vi "3. ControlRealTimeACCESS.vi"() -> ()   [LabVIEW 2011]
panel:
  out "Iteration #":i32
  out "mote111":cluster{dbl, dbl}
  out "mote110":cluster{dbl, dbl}
  out "mote109":cluster{dbl, dbl}
  out "mote12":cluster{dbl, dbl}
  out "mote11":cluster{dbl, dbl}
  out "mote8":cluster{dbl, dbl}
  out "mote7":cluster{dbl, dbl}
  out "mote6":cluster{dbl, dbl}
  out "mote5":cluster{dbl, dbl}
  out "mote3":cluster{dbl, dbl}
  out "mote2":cluster{dbl, dbl}
  out "mote4":cluster{dbl, dbl, dbl, dbl}
  out "mote1":cluster{dbl, dbl, dbl, dbl}
  in  "HVAC Testbed":T1(tab)
  out "Motion":bool
  out "CO2":string
  out "Temp":string
  out "Temp":string
  out "CO2":string
  out "Motion":bool
  out "Temp":string
  out "CO2":string
  out "Motion":bool
  out "CO2":string
  out "Temp":string
  out "Motion":bool
  out "Outside temp":dbl(slide) scale=-20.0..40.0
  in  "Heating Valve":u64(slide) scale=0.0..100.0
  in  "Cooling Valve":u64(slide) scale=0.0..100.0
  in  "Fresh Air Valve":u64(slide) scale=0.0..100.0
  out "Temp":string
  out "CO2":string
  out "Motion":bool
  out "CO2":dbl(graph)
  out "Temperature":dbl(graph)
  out "CO2":dbl(graph)
  out "Temperature":dbl(graph)
  in  "Heating Valve":u64(slide) scale=0.0..100.0
  in  "Cooling Valve":u64(slide) scale=0.0..100.0
  in  "Fresh Air Valve":u64(slide) scale=0.0..100.0
  out "Occupancy":dbl
  out "Temp":string
  out "CO2":string
  out "Motion":bool
  out "Light":dbl(slide) scale=0.0..100.0
  in  "12":bool
  in  "11":bool
  in  "4":bool
  in  "111":bool
  in  "110":bool
  in  "109":bool
  in  "8":bool
  in  "7":bool
  in  "5":bool
  in  "4":bool
  in  "3":bool
  in  "1":bool
  in  "6":bool
  in  "2":bool
  out "Humidity":dbl(slide) scale=0.0..100.0
  out "Temperature":dbl(slide) scale=0.0..100.0
  out "CO2 Meter":dbl(knob) scale=0.0..800.0
  out "Selected Mote":string
  out "CO2":dbl(graph)
  out "Temperature":dbl(graph)
  in  "Heating Valve":u64(slide) scale=0.0..100.0
  in  "Cooling Valve":u64(slide) scale=0.0..100.0
  in  "Fresh Air Valve":u64(slide) scale=0.0..100.0
  out "Temp":string
  out "CO2":string
  out "Motion":bool
  in  "HVAC System IP Address":string(combo)="130.237.50.30"
  in  "Password":string
  in  "Username":string
  out "Access to HVAC Msg":errorcluster={"status"=FALSE, "code"=0, "source"="Please Wait ..."}
  # "Actuation"
  # "PLC Data"
  # "Selected Mote Data"
  # "PLC Data"
  # "Actuation"
  # "Actuation"
  # "PLC Data"
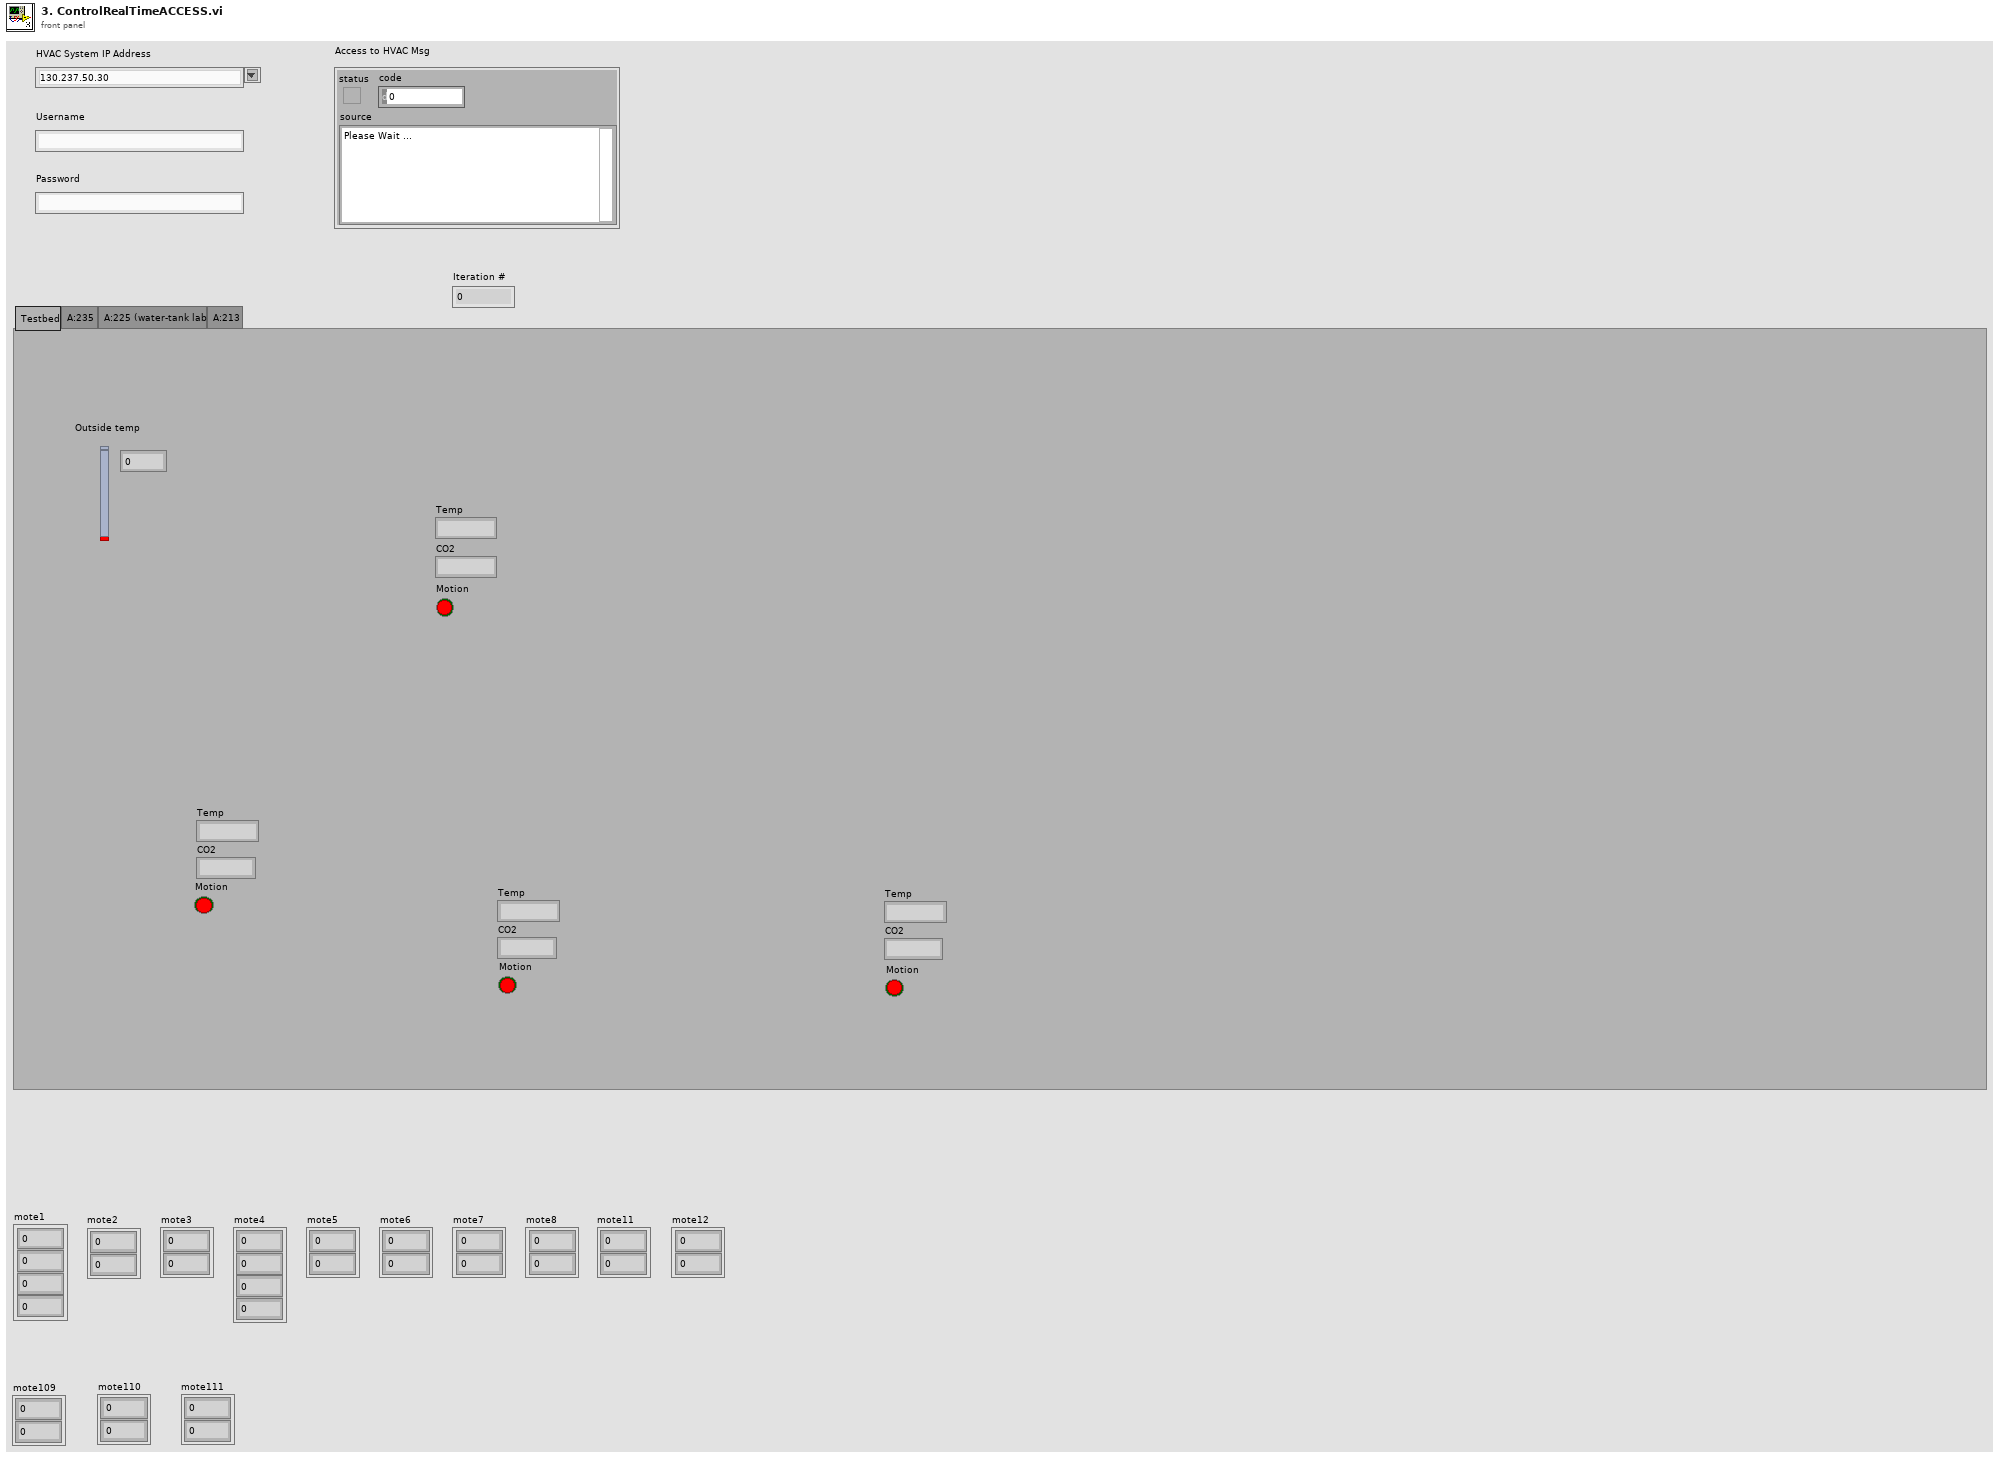
[diagram p1: front panel]
types:
  T1 = enum32{"Testbed", "A:235", "A:225 (water-tank lab)", "A:213"}
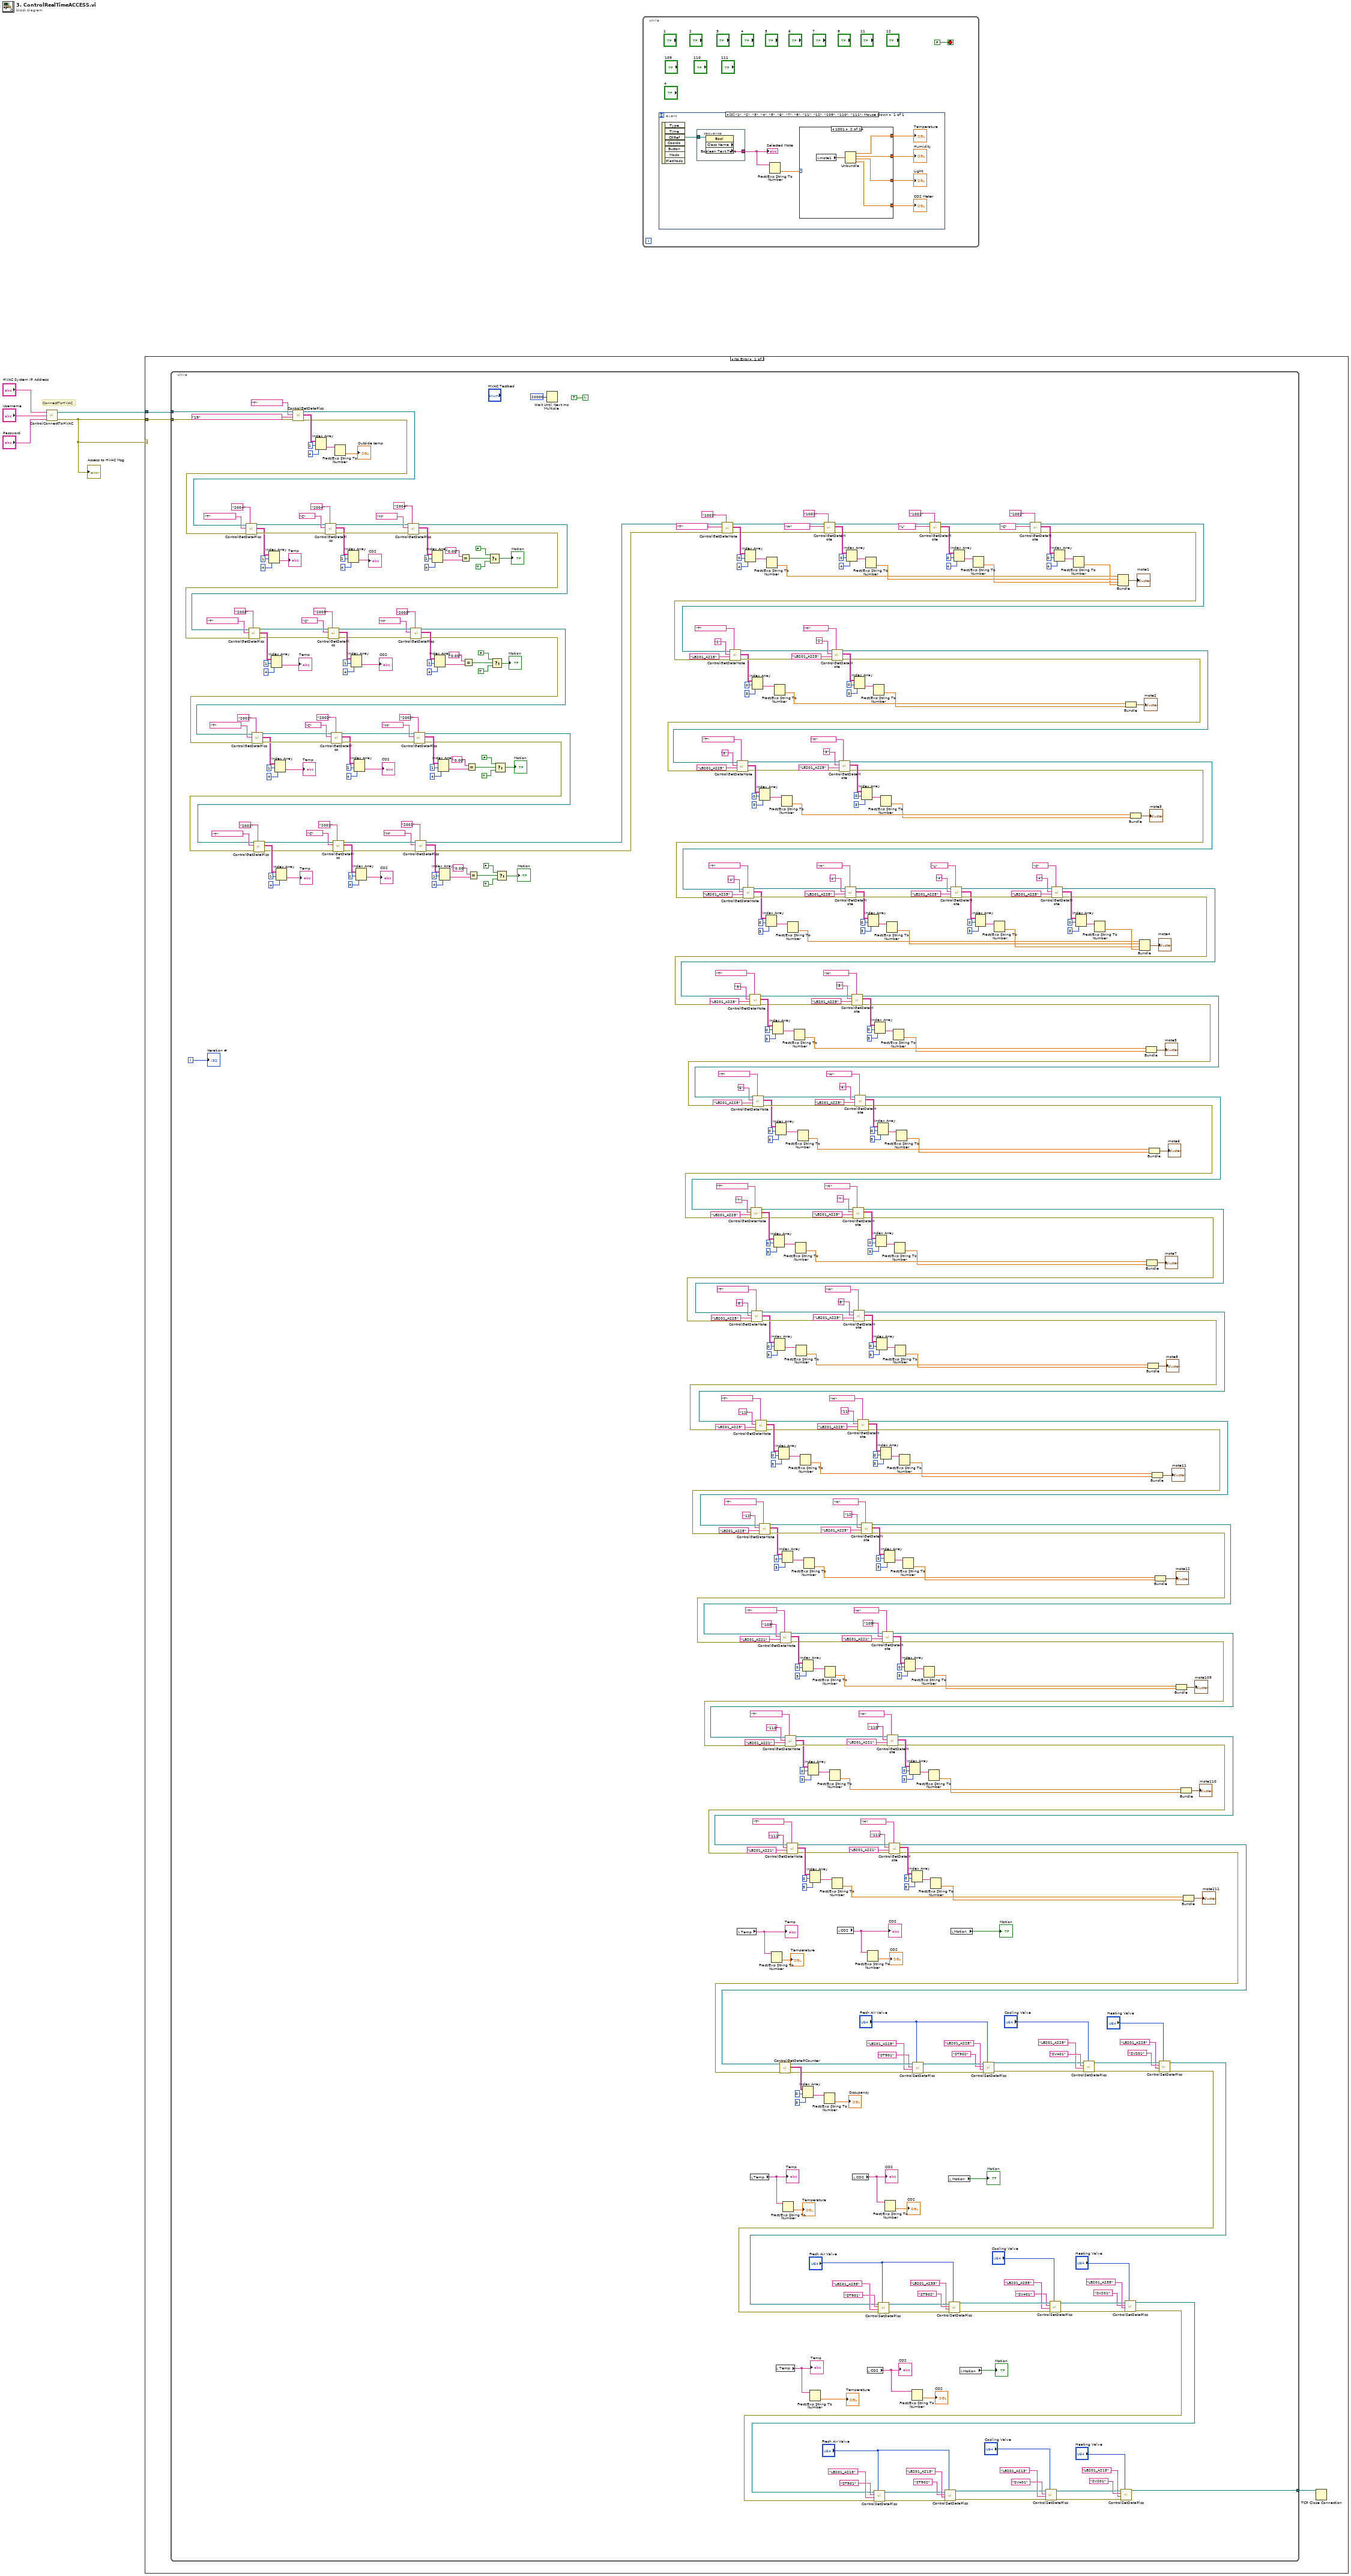
[diagram p0: block diagram]
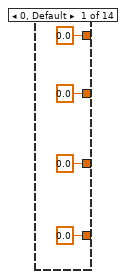
[diagram p2: hidden frame]
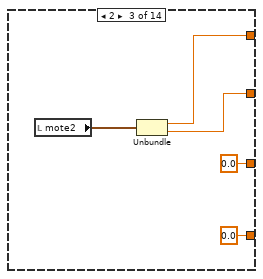
[diagram p3: hidden frame]
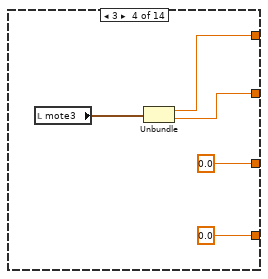
[diagram p4: hidden frame]
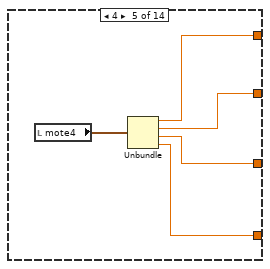
[diagram p5: hidden frame]
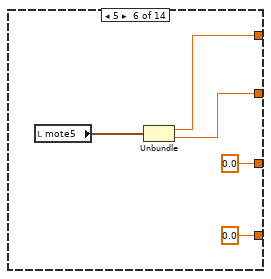
[diagram p6: hidden frame]
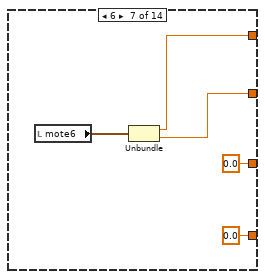
[diagram p7: hidden frame]
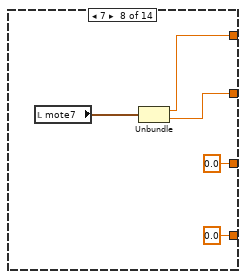
[diagram p8: hidden frame]
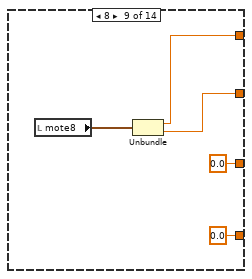
[diagram p9: hidden frame]
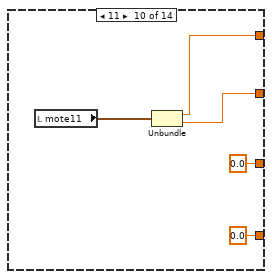
[diagram p10: hidden frame]
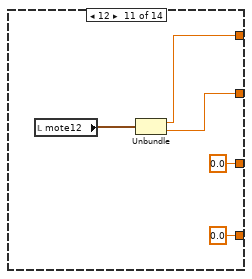
[diagram p11: hidden frame]
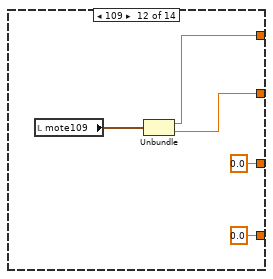
[diagram p12: hidden frame]
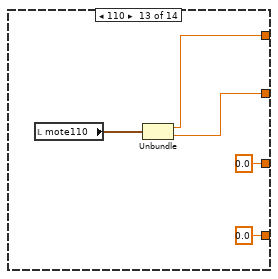
[diagram p13: hidden frame]
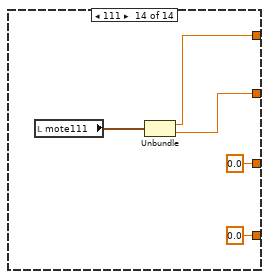
[diagram p14: hidden frame]
diagram:
  # "ConnectToHVAC"
  n1 = call "ControlConnectToHVAC.vi"("Password"="Password", "Username"="Username", "IP Address"="HVAC System IP Address") -> ("error out"=w4:errorcluster, "connection ID out"=w5:refnum<k5>)  [unwired: 1 in]
  "Access to HVAC Msg" <- w4
  n2 = case shown="No Error" w4 {
    tunnel: w5 -> [w7 _]
    tunnel: w4 -> [w8 _]
    frame No Error {
      n3 = while {
        tunnel: w7 -> [w501]
        tunnel: w8 -> [w502]
        tunnel: [w41] -> w6
        i -> [w396]
        stop <- TRUE continue-if-true
        n4 = call "ControlGetDataPlcs.vi"("error in"=w502, "signalID"="19", "dataType"="T" ("Data Type"), "connection ID in"=w501) -> ("error out"=w499:errorcluster, "output array"=w507:string[][], "connection ID out"=w500:refnum<k5>)  [unwired: 4 in]
        n5 = call "ControlGetDataPlcs.vi"("deviceID"="2004", "error in"=w499, "dataType"="T" ("Data Type"), "connection ID in"=w500) -> ("error out"=w519:errorcluster, "output array"=w514:string[][], "connection ID out"=w520:refnum<k5>)  [unwired: 4 in]
        n6 = Index Array(array=w514, index (row)=1, index (col)=4 ("disabled index (col)")) -> (element=→"Temp":string)
        n7 = Index Array(array=w507, index (row)=1, index (col)=4 ("disabled index (col)")) -> (element=w506:string)
        n8 = call "ControlGetDataPlcs.vi"("deviceID"="2004", "error in"=w519, "dataType"="C" ("Data Type"), "connection ID in"=w520) -> ("error out"=w518:errorcluster, "output array"=w509:string[][], "connection ID out"=w517:refnum<k5>)  [unwired: 4 in]
        n9 = Fract/Exp String To Number(string=w506) -> (number=→"Outside temp":dbl)  [unwired: 3 in, 1 out]
        n10 = Index Array(array=w509, index (row)=1, index (col)=4 ("disabled index (col)")) -> (element=→"CO2":string)
        n11 = call "ControlGetDataPlcs.vi"("deviceID"="2004", "error in"=w518, "dataType"="M" ("Data Type"), "connection ID in"=w517) -> ("error out"=w471:errorcluster, "output array"=w508:string[][], "connection ID out"=w472:refnum<k5>)  [unwired: 4 in]
        n12 = call "ControlGetDataPlcs.vi"("deviceID"="2003", "error in"=w471, "dataType"="T" ("Data Type"), "connection ID in"=w472) -> ("error out"=w477:errorcluster, "output array"=w482:string[][], "connection ID out"=w476:refnum<k5>)  [unwired: 4 in]
        n13 = Index Array(array=w482, index (row)=1, index (col)=4 ("disabled index (col)")) -> (element=→"Temp":string)
        n14 = call "ControlGetDataPlcs.vi"("deviceID"="2003", "error in"=w477, "dataType"="C" ("Data Type"), "connection ID in"=w476) -> ("error out"=w478:errorcluster, "output array"=w487:string[][], "connection ID out"=w479:refnum<k5>)  [unwired: 4 in]
        n15 = Index Array(array=w487, index (row)=1, index (col)=4 ("disabled index (col)")) -> (element=→"CO2":string)
        n16 = call "ControlGetDataPlcs.vi"("deviceID"="2003", "error in"=w478, "dataType"="M" ("Data Type"), "connection ID in"=w479) -> ("error out"=w448:errorcluster, "output array"=w488:string[][], "connection ID out"=w449:refnum<k5>)  [unwired: 4 in]
        n17 = call "ControlGetDataPlcs.vi"("deviceID"="2002", "error in"=w448, "dataType"="T" ("Data Type"), "connection ID in"=w449) -> ("error out"=w466:errorcluster, "output array"=w461:string[][], "connection ID out"=w467:refnum<k5>)  [unwired: 4 in]
        n18 = Index Array(array=w461, index (row)=1, index (col)=4 ("disabled index (col)")) -> (element=→"Temp":string)
        n19 = call "ControlGetDataPlcs.vi"("deviceID"="2002", "error in"=w466, "dataType"="C" ("Data Type"), "connection ID in"=w467) -> ("error out"=w465:errorcluster, "output array"=w456:string[][], "connection ID out"=w464:refnum<k5>)  [unwired: 4 in]
        n20 = Index Array(array=w456, index (row)=1, index (col)=4 ("disabled index (col)")) -> (element=→"CO2":string)
        n21 = call "ControlGetDataPlcs.vi"("deviceID"="2002", "error in"=w465, "dataType"="M" ("Data Type"), "connection ID in"=w464) -> ("error out"=w425:errorcluster, "output array"=w455:string[][], "connection ID out"=w426:refnum<k5>)  [unwired: 4 in]
        n22 = call "ControlGetDataPlcs.vi"("deviceID"="2001", "error in"=w425, "dataType"="T" ("Data Type"), "connection ID in"=w426) -> ("error out"=w431:errorcluster, "output array"=w436:string[][], "connection ID out"=w430:refnum<k5>)  [unwired: 4 in]
        n23 = Index Array(array=w436, index (row)=1, index (col)=4 ("disabled index (col)")) -> (element=→"Temp":string)
        n24 = call "ControlGetDataPlcs.vi"("deviceID"="2001", "error in"=w431, "dataType"="C" ("Data Type"), "connection ID in"=w430) -> ("error out"=w432:errorcluster, "output array"=w441:string[][], "connection ID out"=w433:refnum<k5>)  [unwired: 4 in]
        n25 = Index Array(array=w441, index (row)=1, index (col)=4 ("disabled index (col)")) -> (element=→"CO2":string)
        n26 = call "ControlGetDataPlcs.vi"("deviceID"="2001", "error in"=w432, "dataType"="M" ("Data Type"), "connection ID in"=w433) -> ("error out"=w397:errorcluster, "output array"=w442:string[][], "connection ID out"=w398:refnum<k5>)  [unwired: 4 in]
        n27 = Index Array(array=w508, index (row)=1, index (col)=4 ("disabled index (col)")) -> (element=w497:string)
        n28 = Index Array(array=w488, index (row)=1, index (col)=4 ("disabled index (col)")) -> (element=w490:string)
        n29 = Index Array(array=w455, index (row)=1, index (col)=4 ("disabled index (col)")) -> (element=w453:string)
        n30 = Index Array(array=w442, index (row)=1, index (col)=4 ("disabled index (col)")) -> (element=w444:string)
        n31 = Equal?(x="0.00", y=w497) -> (x = y?=w496:bool)
        n32 = Equal?(x="0.00", y=w490) -> (x = y?=w491:bool)
        n33 = Equal?(x="0.00", y=w453) -> (x = y?=w452:bool)
        n34 = Equal?(x="0.00", y=w444) -> (x = y?=w445:bool)
        n35 = Select(t=FALSE, s=w496, f=TRUE) -> (s? t:f=→"Motion":bool)
        n36 = Select(t=FALSE, s=w491, f=TRUE) -> (s? t:f=→"Motion":bool)
        n37 = Select(t=FALSE, s=w452, f=TRUE) -> (s? t:f=→"Motion":bool)
        n38 = Select(t=FALSE, s=w445, f=TRUE) -> (s? t:f=→"Motion":bool)
        n39 = Wait Until Next ms Multiple(millisecond multiple=u32 20000) -> ()  [unwired: 1 out]
        n40 = call "ControlGetDataMote.vi"("deviceID"="1001" ("Node ID"), "error in"=w397, "dataType"="T" ("Data Type"), "connection ID in"=w398) -> ("error out"=w400:errorcluster, "output array"=w405:string[][], "connection ID out"=w399:refnum<k5>)  [unwired: 5 in]
        n41 = local read "Temp"() -> (w83:string)
        "Temp" <- w83
        n42 = Index Array(array=w405, index (row)=0, index (col)=4 ("disabled index (col)")) -> (element=w395:string)
        n43 = local read "Temp"() -> (w78:string)
        "Temp" <- w78
        n44 = Fract/Exp String To Number(string=w395) -> (number=w392:dbl)  [unwired: 3 in, 1 out]
        n45 = Fract/Exp String To Number(string=w83) -> (number=→"Temperature":dbl)  [unwired: 3 in, 1 out]
        n46 = local read "Temp"() -> (w59:string)
        "Temp" <- w59
        n47 = Fract/Exp String To Number(string=w78) -> (number=→"Temperature":dbl)  [unwired: 3 in, 1 out]
        n48 = Fract/Exp String To Number(string=w59) -> (number=→"Temperature":dbl)  [unwired: 3 in, 1 out]
        n49 = call "ControlGetDataMote.vi"("deviceID"="1001" ("Node ID"), "error in"=w400, "dataType"="H" ("Data Type"), "connection ID in"=w399) -> ("error out"=w401:errorcluster, "output array"=w410:string[][], "connection ID out"=w402:refnum<k5>)  [unwired: 5 in]
        n50 = local read "CO2"() -> (w82:string)
        "CO2" <- w82
        n51 = Index Array(array=w410, index (row)=0, index (col)=4 ("disabled index (col)")) -> (element=w394:string)
        n52 = local read "CO2"() -> (w77:string)
        "CO2" <- w77
        n53 = Fract/Exp String To Number(string=w394) -> (number=w391:dbl)  [unwired: 3 in, 1 out]
        n54 = Fract/Exp String To Number(string=w82) -> (number=→"CO2":dbl)  [unwired: 3 in, 1 out]
        n55 = local read "CO2"() -> (w58:string)
        "CO2" <- w58
        n56 = Fract/Exp String To Number(string=w77) -> (number=→"CO2":dbl)  [unwired: 3 in, 1 out]
        n57 = Fract/Exp String To Number(string=w58) -> (number=→"CO2":dbl)  [unwired: 3 in, 1 out]
        n58 = call "ControlGetDataMote.vi"("deviceID"="1001" ("Node ID"), "error in"=w401, "dataType"="L" ("Data Type"), "connection ID in"=w402) -> ("error out"=w382:errorcluster, "output array"=w411:string[][], "connection ID out"=w385:refnum<k5>)  [unwired: 5 in]
        n59 = local read "Motion"() -> (→"Motion":bool)
        n60 = local read "Motion"() -> (→"Motion":bool)
        n61 = Index Array(array=w411, index (row)=0, index (col)=4 ("disabled index (col)")) -> (element=w393:string)
        n62 = local read "Motion"() -> (→"Motion":bool)
        n63 = Fract/Exp String To Number(string=w393) -> (number=w390:dbl)  [unwired: 3 in, 1 out]
        n64 = call "ControlGetDataMote.vi"("deviceID"="1001" ("Node ID"), "error in"=w382, "dataType"="C" ("Data Type"), "connection ID in"=w385) -> ("error out"=w305:errorcluster, "output array"=w386:string[][], "connection ID out"=w306:refnum<k5>)  [unwired: 5 in]
        n65 = call "ControlGetDataMote.vi"("deviceID"="T" ("Data Type"), "error in"=w305, "signalID"="LB201_A225" ("Location"), "dataType"="2" ("Node ID"), "connection ID in"=w306) -> ("error out"=w370:errorcluster, "output array"=w367:string[][], "connection ID out"=w371:refnum<k5>)  [unwired: 4 in]
        n66 = Index Array(array=w367, index (row)=0, index (col)=3 ("disabled index (col)")) -> (element=w378:string)
        n67 = Fract/Exp String To Number(string=w378) -> (number=w380:dbl)  [unwired: 3 in, 1 out]
        n68 = call "ControlGetDataMote.vi"("deviceID"="H" ("Data Type"), "error in"=w370, "signalID"="LB201_A225" ("Location"), "dataType"="2" ("Node ID"), "connection ID in"=w371) -> ("error out"=w301:errorcluster, "output array"=w364:string[][], "connection ID out"=w302:refnum<k5>)  [unwired: 4 in]
        n69 = call "ControlGetDataMote.vi"("deviceID"="T" ("Data Type"), "error in"=w301, "signalID"="LB201_A225" ("Location"), "dataType"="3" ("Node ID"), "connection ID in"=w302) -> ("error out"=w357:errorcluster, "output array"=w360:string[][], "connection ID out"=w356:refnum<k5>)  [unwired: 4 in]
        n70 = Index Array(array=w360, index (row)=0, index (col)=3 ("disabled index (col)")) -> (element=w349:string)
        n71 = Fract/Exp String To Number(string=w349) -> (number=w347:dbl)  [unwired: 3 in, 1 out]
        n72 = call "ControlGetDataMote.vi"("deviceID"="H" ("Data Type"), "error in"=w357, "signalID"="LB201_A225" ("Location"), "dataType"="3" ("Node ID"), "connection ID in"=w356) -> ("error out"=w303:errorcluster, "output array"=w363:string[][], "connection ID out"=w304:refnum<k5>)  [unwired: 4 in]
        n73 = call "ControlGetDataMote.vi"("deviceID"="T" ("Data Type"), "error in"=w303, "signalID"="LB201_A225" ("Location"), "dataType"="4" ("Node ID"), "connection ID in"=w304) -> ("error out"=w318:errorcluster, "output array"=w313:string[][], "connection ID out"=w319:refnum<k5>)  [unwired: 4 in]
        n74 = Index Array(array=w313, index (row)=0, index (col)=3 ("disabled index (col)")) -> (element=w329:string)
        n75 = Fract/Exp String To Number(string=w329) -> (number=w332:dbl)  [unwired: 3 in, 1 out]
        n76 = call "ControlGetDataMote.vi"("deviceID"="H" ("Data Type"), "error in"=w318, "signalID"="LB201_A225" ("Location"), "dataType"="4" ("Node ID"), "connection ID in"=w319) -> ("error out"=w317:errorcluster, "output array"=w308:string[][], "connection ID out"=w316:refnum<k5>)  [unwired: 4 in]
        n77 = Index Array(array=w364, index (row)=0, index (col)=3 ("disabled index (col)")) -> (element=w379:string)
        n78 = Index Array(array=w363, index (row)=0, index (col)=3 ("disabled index (col)")) -> (element=w348:string)
        n79 = Index Array(array=w308, index (row)=0, index (col)=3 ("disabled index (col)")) -> (element=w330:string)
        n80 = Fract/Exp String To Number(string=w379) -> (number=w381:dbl)  [unwired: 3 in, 1 out]
        n81 = Fract/Exp String To Number(string=w348) -> (number=w346:dbl)  [unwired: 3 in, 1 out]
        n82 = Fract/Exp String To Number(string=w330) -> (number=w333:dbl)  [unwired: 3 in, 1 out]
        n83 = call "ControlGetDataMote.vi"("deviceID"="L" ("Data Type"), "error in"=w317, "signalID"="LB201_A225" ("Location"), "dataType"="4" ("Node ID"), "connection ID in"=w316) -> ("error out"=w345:errorcluster, "output array"=w307:string[][], "connection ID out"=w342:refnum<k5>)  [unwired: 4 in]
        n84 = Index Array(array=w307, index (row)=0, index (col)=3 ("disabled index (col)")) -> (element=w331:string)
        n85 = Fract/Exp String To Number(string=w331) -> (number=w334:dbl)  [unwired: 3 in, 1 out]
        n86 = call "ControlGetDataMote.vi"("deviceID"="C" ("Data Type"), "error in"=w345, "signalID"="LB201_A225" ("Location"), "dataType"="4" ("Node ID"), "connection ID in"=w342) -> ("error out"=w189:errorcluster, "output array"=w341:string[][], "connection ID out"=w190:refnum<k5>)  [unwired: 4 in]
        n87 = call "ControlGetDataMote.vi"("deviceID"="T" ("Data Type"), "error in"=w189, "signalID"="LB201_A225" ("Location"), "dataType"="5" ("Node ID"), "connection ID in"=w190) -> ("error out"=w292:errorcluster, "output array"=w295:string[][], "connection ID out"=w291:refnum<k5>)  [unwired: 4 in]
        n88 = Index Array(array=w295, index (row)=0, index (col)=3 ("disabled index (col)")) -> (element=w284:string)
        n89 = Fract/Exp String To Number(string=w284) -> (number=w282:dbl)  [unwired: 3 in, 1 out]
        n90 = call "ControlGetDataMote.vi"("deviceID"="H" ("Data Type"), "error in"=w292, "signalID"="LB201_A225" ("Location"), "dataType"="5" ("Node ID"), "connection ID in"=w291) -> ("error out"=w185:errorcluster, "output array"=w298:string[][], "connection ID out"=w186:refnum<k5>)  [unwired: 4 in]
        n91 = call "ControlGetDataMote.vi"("deviceID"="T" ("Data Type"), "error in"=w185, "signalID"="LB201_A225" ("Location"), "dataType"="6" ("Node ID"), "connection ID in"=w186) -> ("error out"=w269:errorcluster, "output array"=w266:string[][], "connection ID out"=w270:refnum<k5>)  [unwired: 4 in]
        n92 = Index Array(array=w266, index (row)=0, index (col)=3 ("disabled index (col)")) -> (element=w277:string)
        n93 = Fract/Exp String To Number(string=w277) -> (number=w279:dbl)  [unwired: 3 in, 1 out]
        n94 = call "ControlGetDataMote.vi"("deviceID"="H" ("Data Type"), "error in"=w269, "signalID"="LB201_A225" ("Location"), "dataType"="6" ("Node ID"), "connection ID in"=w270) -> ("error out"=w182:errorcluster, "output array"=w263:string[][], "connection ID out"=w183:refnum<k5>)  [unwired: 4 in]
        n95 = call "ControlGetDataMote.vi"("deviceID"="T" ("Data Type"), "error in"=w182, "signalID"="LB201_A225" ("Location"), "dataType"="7" ("Node ID"), "connection ID in"=w183) -> ("error out"=w256:errorcluster, "output array"=w259:string[][], "connection ID out"=w255:refnum<k5>)  [unwired: 4 in]
        n96 = Index Array(array=w259, index (row)=0, index (col)=3 ("disabled index (col)")) -> (element=w248:string)
        n97 = Fract/Exp String To Number(string=w248) -> (number=w246:dbl)  [unwired: 3 in, 1 out]
        n98 = call "ControlGetDataMote.vi"("deviceID"="H" ("Data Type"), "error in"=w256, "signalID"="LB201_A225" ("Location"), "dataType"="7" ("Node ID"), "connection ID in"=w255) -> ("error out"=w179:errorcluster, "output array"=w262:string[][], "connection ID out"=w180:refnum<k5>)  [unwired: 4 in]
        n99 = call "ControlGetDataMote.vi"("deviceID"="T" ("Data Type"), "error in"=w179, "signalID"="LB201_A225" ("Location"), "dataType"="8" ("Node ID"), "connection ID in"=w180) -> ("error out"=w233:errorcluster, "output array"=w230:string[][], "connection ID out"=w234:refnum<k5>)  [unwired: 4 in]
        n100 = Index Array(array=w230, index (row)=0, index (col)=3 ("disabled index (col)")) -> (element=w241:string)
        n101 = Fract/Exp String To Number(string=w241) -> (number=w243:dbl)  [unwired: 3 in, 1 out]
        n102 = call "ControlGetDataMote.vi"("deviceID"="H" ("Data Type"), "error in"=w233, "signalID"="LB201_A225" ("Location"), "dataType"="8" ("Node ID"), "connection ID in"=w234) -> ("error out"=w139:errorcluster, "output array"=w227:string[][], "connection ID out"=w140:refnum<k5>)  [unwired: 4 in]
        n103 = call "ControlGetDataMote.vi"("deviceID"="T" ("Data Type"), "error in"=w139, "signalID"="LB201_A225" ("Location"), "dataType"="11" ("Node ID"), "connection ID in"=w140) -> ("error out"=w220:errorcluster, "output array"=w223:string[][], "connection ID out"=w219:refnum<k5>)  [unwired: 4 in]
        n104 = Index Array(array=w223, index (row)=0, index (col)=3 ("disabled index (col)")) -> (element=w212:string)
        n105 = Fract/Exp String To Number(string=w212) -> (number=w210:dbl)  [unwired: 3 in, 1 out]
        n106 = call "ControlGetDataMote.vi"("deviceID"="H" ("Data Type"), "error in"=w220, "signalID"="LB201_A225" ("Location"), "dataType"="11" ("Node ID"), "connection ID in"=w219) -> ("error out"=w137:errorcluster, "output array"=w226:string[][], "connection ID out"=w138:refnum<k5>)  [unwired: 4 in]
        n107 = call "ControlGetDataMote.vi"("deviceID"="T" ("Data Type"), "error in"=w137, "signalID"="LB201_A225" ("Location"), "dataType"="12" ("Node ID"), "connection ID in"=w138) -> ("error out"=w197:errorcluster, "output array"=w194:string[][], "connection ID out"=w198:refnum<k5>)  [unwired: 4 in]
        n108 = Index Array(array=w194, index (row)=0, index (col)=3 ("disabled index (col)")) -> (element=w205:string)
        n109 = Fract/Exp String To Number(string=w205) -> (number=w207:dbl)  [unwired: 3 in, 1 out]
        n110 = call "ControlGetDataMote.vi"("deviceID"="H" ("Data Type"), "error in"=w197, "signalID"="LB201_A225" ("Location"), "dataType"="12" ("Node ID"), "connection ID in"=w198) -> ("error out"=w114:errorcluster, "output array"=w191:string[][], "connection ID out"=w115:refnum<k5>)  [unwired: 4 in]
        n111 = call "ControlGetDataMote.vi"("deviceID"="T" ("Data Type"), "error in"=w114, "signalID"="LB201_A221" ("Location"), "dataType"="109" ("Node ID"), "connection ID in"=w115) -> ("error out"=w172:errorcluster, "output array"=w175:string[][], "connection ID out"=w171:refnum<k5>)  [unwired: 4 in]
        n112 = Index Array(array=w175, index (row)=0, index (col)=3 ("disabled index (col)")) -> (element=w164:string)
        n113 = Fract/Exp String To Number(string=w164) -> (number=w162:dbl)  [unwired: 3 in, 1 out]
        n114 = Index Array(array=w298, index (row)=0, index (col)=3 ("disabled index (col)")) -> (element=w283:string)
        n115 = Index Array(array=w262, index (row)=0, index (col)=3 ("disabled index (col)")) -> (element=w247:string)
        n116 = Index Array(array=w227, index (row)=0, index (col)=3 ("disabled index (col)")) -> (element=w242:string)
        n117 = Index Array(array=w263, index (row)=0, index (col)=3 ("disabled index (col)")) -> (element=w278:string)
        n118 = Index Array(array=w226, index (row)=0, index (col)=3 ("disabled index (col)")) -> (element=w211:string)
        n119 = call "ControlGetDataMote.vi"("deviceID"="H" ("Data Type"), "error in"=w172, "signalID"="LB201_A221" ("Location"), "dataType"="109" ("Node ID"), "connection ID in"=w171) -> ("error out"=w112:errorcluster, "output array"=w178:string[][], "connection ID out"=w113:refnum<k5>)  [unwired: 4 in]
        n120 = call "ControlGetDataMote.vi"("deviceID"="T" ("Data Type"), "error in"=w112, "signalID"="LB201_A221" ("Location"), "dataType"="110" ("Node ID"), "connection ID in"=w113) -> ("error out"=w149:errorcluster, "output array"=w146:string[][], "connection ID out"=w150:refnum<k5>)  [unwired: 4 in]
        n121 = Index Array(array=w146, index (row)=0, index (col)=3 ("disabled index (col)")) -> (element=w157:string)
        n122 = Fract/Exp String To Number(string=w157) -> (number=w159:dbl)  [unwired: 3 in, 1 out]
        n123 = Index Array(array=w191, index (row)=0, index (col)=3 ("disabled index (col)")) -> (element=w206:string)
        n124 = call "ControlGetDataMote.vi"("deviceID"="H" ("Data Type"), "error in"=w149, "signalID"="LB201_A221" ("Location"), "dataType"="110" ("Node ID"), "connection ID in"=w150) -> ("error out"=w110:errorcluster, "output array"=w143:string[][], "connection ID out"=w111:refnum<k5>)  [unwired: 4 in]
        n125 = call "ControlGetDataMote.vi"("deviceID"="T" ("Data Type"), "error in"=w110, "signalID"="LB201_A221" ("Location"), "dataType"="111" ("Node ID"), "connection ID in"=w111) -> ("error out"=w130:errorcluster, "output array"=w133:string[][], "connection ID out"=w129:refnum<k5>)  [unwired: 4 in]
        n126 = Index Array(array=w133, index (row)=0, index (col)=3 ("disabled index (col)")) -> (element=w122:string)
        n127 = Fract/Exp String To Number(string=w122) -> (number=w120:dbl)  [unwired: 3 in, 1 out]
        n128 = call "ControlGetDataMote.vi"("deviceID"="H" ("Data Type"), "error in"=w130, "signalID"="LB201_A221" ("Location"), "dataType"="111" ("Node ID"), "connection ID in"=w129) -> ("error out"=w104:errorcluster, "output array"=w136:string[][], "connection ID out"=w102:refnum<k5>)  [unwired: 4 in]
        n129 = call "ControlGetDataPCounter.vi"("error in"=w104, "connection ID in"=w102) -> ("error out"=w100:errorcluster, "output array"=w105:string[][], "connection ID out"=w101:refnum<k5>)  [unwired: 7 in]
        n130 = Index Array(array=w105, index (row)=0, index (col)=3 ("disabled index (col)")) -> (element=w108:string)
        n131 = Fract/Exp String To Number(string=w108) -> (number=→"Occupancy":dbl)  [unwired: 3 in, 1 out]
        n132 = Fract/Exp String To Number(string=w283) -> (number=w281:dbl)  [unwired: 3 in, 1 out]
        n133 = Fract/Exp String To Number(string=w247) -> (number=w245:dbl)  [unwired: 3 in, 1 out]
        n134 = Fract/Exp String To Number(string=w242) -> (number=w244:dbl)  [unwired: 3 in, 1 out]
        n135 = Fract/Exp String To Number(string=w278) -> (number=w280:dbl)  [unwired: 3 in, 1 out]
        n136 = Fract/Exp String To Number(string=w211) -> (number=w209:dbl)  [unwired: 3 in, 1 out]
        n137 = Fract/Exp String To Number(string=w206) -> (number=w208:dbl)  [unwired: 3 in, 1 out]
        n138 = Index Array(array=w178, index (row)=0, index (col)=3 ("disabled index (col)")) -> (element=w163:string)
        n139 = Index Array(array=w143, index (row)=0, index (col)=3 ("disabled index (col)")) -> (element=w158:string)
        n140 = Index Array(array=w136, index (row)=0, index (col)=3 ("disabled index (col)")) -> (element=w121:string)
        n141 = call "ControlSetDataPlcs.vi"("data"="Fresh Air Valve", "error in"=w100, "location"="LB201_A225" ("Location"), "signalID"="ST901" ("Node ID"), "connection ID in"=w101) -> ("error out"=w96:errorcluster, "connection ID out"=w97:refnum<k5>)  [unwired: 3 in, 1 out]
        n142 = Fract/Exp String To Number(string=w163) -> (number=w161:dbl)  [unwired: 3 in, 1 out]
        n143 = Fract/Exp String To Number(string=w158) -> (number=w160:dbl)  [unwired: 3 in, 1 out]
        n144 = Fract/Exp String To Number(string=w121) -> (number=w119:dbl)  [unwired: 3 in, 1 out]
        n145 = call "ControlSetDataPlcs.vi"("data"="Fresh Air Valve", "error in"=w96, "location"="LB201_A225" ("Location"), "signalID"="ST902" ("Node ID"), "connection ID in"=w97) -> ("error out"=w86:errorcluster, "connection ID out"=w87:refnum<k5>)  [unwired: 3 in, 1 out]
        n146 = Index Array(array=w386, index (row)=0, index (col)=4 ("disabled index (col)")) -> (element=w389:string)
        n147 = Fract/Exp String To Number(string=w389) -> (number=w384:dbl)  [unwired: 3 in, 1 out]
        n148 = Index Array(array=w341, index (row)=0, index (col)=3 ("disabled index (col)")) -> (element=w335:string)
        n149 = call "ControlSetDataPlcs.vi"("data"="Cooling Valve", "error in"=w86, "location"="LB201_A225" ("Location"), "signalID"="SV401" ("Node ID"), "connection ID in"=w87) -> ("error out"=w91:errorcluster, "connection ID out"=w90:refnum<k5>)  [unwired: 3 in, 1 out]
        n150 = Fract/Exp String To Number(string=w335) -> (number=w343:dbl)  [unwired: 3 in, 1 out]
        n151 = Bundle(w392, w391, w390, w384) -> (→"mote1":cluster{dbl, dbl, dbl, dbl})  [unwired: 1 in]
        n152 = Bundle(w380, w381) -> (→"mote2":cluster{dbl, dbl})  [unwired: 1 in]
        n153 = Bundle(w347, w346) -> (→"mote3":cluster{dbl, dbl})  [unwired: 1 in]
        n154 = Bundle(w332, w333, w334, w343) -> (→"mote4":cluster{dbl, dbl, dbl, dbl})  [unwired: 1 in]
        n155 = Bundle(w282, w281) -> (→"mote5":cluster{dbl, dbl})  [unwired: 1 in]
        n156 = Bundle(w246, w245) -> (→"mote7":cluster{dbl, dbl})  [unwired: 1 in]
        n157 = Bundle(w243, w244) -> (→"mote8":cluster{dbl, dbl})  [unwired: 1 in]
        n158 = Bundle(w279, w280) -> (→"mote6":cluster{dbl, dbl})  [unwired: 1 in]
        n159 = Bundle(w210, w209) -> (→"mote11":cluster{dbl, dbl})  [unwired: 1 in]
        n160 = Bundle(w207, w208) -> (→"mote12":cluster{dbl, dbl})  [unwired: 1 in]
        n161 = call "ControlSetDataPlcs.vi"("data"="Heating Valve", "error in"=w91, "location"="LB201_A225" ("Location"), "signalID"="SV201" ("Node ID"), "connection ID in"=w90) -> ("error out"=w61:errorcluster, "connection ID out"=w62:refnum<k5>)  [unwired: 3 in, 1 out]
        n162 = call "ControlSetDataPlcs.vi"("data"="Fresh Air Valve", "error in"=w61, "location"="LB201_A235" ("Location"), "signalID"="ST901" ("Node ID"), "connection ID in"=w62) -> ("error out"=w66:errorcluster, "connection ID out"=w65:refnum<k5>)  [unwired: 3 in, 1 out]
        n163 = call "ControlSetDataPlcs.vi"("data"="Fresh Air Valve", "error in"=w66, "location"="LB201_A235" ("Location"), "signalID"="ST902" ("Node ID"), "connection ID in"=w65) -> ("error out"=w76:errorcluster, "connection ID out"=w75:refnum<k5>)  [unwired: 3 in, 1 out]
        n164 = call "ControlSetDataPlcs.vi"("data"="Cooling Valve", "error in"=w76, "location"="LB201_A235" ("Location"), "signalID"="SV401" ("Node ID"), "connection ID in"=w75) -> ("error out"=w71:errorcluster, "connection ID out"=w72:refnum<k5>)  [unwired: 3 in, 1 out]
        n165 = call "ControlSetDataPlcs.vi"("data"="Heating Valve", "error in"=w71, "location"="LB201_A235" ("Location"), "signalID"="SV201" ("Node ID"), "connection ID in"=w72) -> ("error out"=w42:errorcluster, "connection ID out"=w43:refnum<k5>)  [unwired: 3 in, 1 out]
        n166 = call "ControlSetDataPlcs.vi"("data"="Fresh Air Valve", "error in"=w42, "location"="LB201_A213" ("Location"), "signalID"="ST901" ("Node ID"), "connection ID in"=w43) -> ("error out"=w54:errorcluster, "connection ID out"=w55:refnum<k5>)  [unwired: 3 in, 1 out]
        n167 = call "ControlSetDataPlcs.vi"("data"="Fresh Air Valve", "error in"=w54, "location"="LB201_A213" ("Location"), "signalID"="ST902" ("Node ID"), "connection ID in"=w55) -> ("error out"=w44:errorcluster, "connection ID out"=w45:refnum<k5>)  [unwired: 3 in, 1 out]
        n168 = call "ControlSetDataPlcs.vi"("data"="Cooling Valve", "error in"=w44, "location"="LB201_A213" ("Location"), "signalID"="SV401" ("Node ID"), "connection ID in"=w45) -> ("error out"=w49:errorcluster, "connection ID out"=w48:refnum<k5>)  [unwired: 3 in, 1 out]
        n169 = call "ControlSetDataPlcs.vi"("data"="Heating Valve", "error in"=w49, "location"="LB201_A213" ("Location"), "signalID"="SV201" ("Node ID"), "connection ID in"=w48) -> ("connection ID out"=w41:refnum<k5>)  [unwired: 3 in, 2 out]
        n170 = Bundle(w162, w161) -> (→"mote109":cluster{dbl, dbl})  [unwired: 1 in]
        n171 = Bundle(w159, w160) -> (→"mote110":cluster{dbl, dbl})  [unwired: 1 in]
        n172 = Bundle(w120, w119) -> (→"mote111":cluster{dbl, dbl})  [unwired: 1 in]
        "Iteration #" <- w396
      }
      n173 = TCP Close Connection(connection ID=w6) -> ()  [unwired: 2 in, 2 out]
    }
    frame Error {
    }
  }
  n174 = while {
    stop <- FALSE stop-if-true
    n175 = event shown="[0] \"1\", \"2\", \"3\", \"4\", \"5\", \"6\", \"7\", \"8\", \"11\", \"12\", \"109\", \"110\", \"111\": Mouse Down" {
      selector: _ -> [_]
      dyn-events: _ -> [_]
      timeout: _ -> [_]
      event "1", "2", "3", "4", "5", "6", "7", "8", "11", "12", "109", "110", "111": Mouse Down {
        n176 = event-data() -> ("CtlRef"=w533:refnum<vi>)  [unwired: 1 in, 6 out]
        n177 = stacked-sequence {
          tunnel: [w604] -> w530
          tunnel: w533 -> [w603]
          frame #0 {
            n178 = property class="Bool" props=["Class Name", "Boolean Text", "Text"](reference=w603) -> ("Boolean Text.Text"=w604:string)  [unwired: 1 in, 3 out]
          }
        }
        "Selected Mote" <- w530
        n179 = Fract/Exp String To Number(string=w530) -> (number=w529:dbl)  [unwired: 3 in, 1 out]
        n180 = case shown="1001" w529 {
          tunnel: [0.0 w542 w546 w551 w556 w561 w566 w571 w576 w581 w586 w591 w596 w601] -> w532
          tunnel: [0.0 w541 w545 w550 w555 w560 w565 w570 w575 w580 w585 w590 w595 w600] -> w531
          tunnel: [0.0 w538 0.0 0.0 w553 0.0 0.0 0.0 0.0 0.0 0.0 0.0 0.0 0.0] -> w528
          tunnel: [0.0 w539 0.0 0.0 w554 0.0 0.0 0.0 0.0 0.0 0.0 0.0 0.0 0.0] -> w527
          frame 0, Default {
          }
          frame 1001 {
            n181 = local read "mote1"() -> (w540:cluster{dbl, dbl, dbl, dbl})
            n182 = Unbundle(w540) -> (w542:dbl, w541:dbl, w539:dbl, w538:dbl)
          }
          frame 2 {
            n183 = local read "mote2"() -> (w547:cluster{dbl, dbl})
            n184 = Unbundle(w547) -> (w546:dbl, w545:dbl)
          }
          frame 3 {
            n185 = local read "mote3"() -> (w552:cluster{dbl, dbl})
            n186 = Unbundle(w552) -> (w551:dbl, w550:dbl)
          }
          frame 4 {
            n187 = local read "mote4"() -> (w557:cluster{dbl, dbl, dbl, dbl})
            n188 = Unbundle(w557) -> (w556:dbl, w555:dbl, w554:dbl, w553:dbl)
          }
          frame 5 {
            n189 = local read "mote5"() -> (w562:cluster{dbl, dbl})
            n190 = Unbundle(w562) -> (w561:dbl, w560:dbl)
          }
          frame 6 {
            n191 = local read "mote6"() -> (w567:cluster{dbl, dbl})
            n192 = Unbundle(w567) -> (w566:dbl, w565:dbl)
          }
          frame 7 {
            n193 = local read "mote7"() -> (w572:cluster{dbl, dbl})
            n194 = Unbundle(w572) -> (w571:dbl, w570:dbl)
          }
          frame 8 {
            n195 = local read "mote8"() -> (w577:cluster{dbl, dbl})
            n196 = Unbundle(w577) -> (w576:dbl, w575:dbl)
          }
          frame 11 {
            n197 = local read "mote11"() -> (w582:cluster{dbl, dbl})
            n198 = Unbundle(w582) -> (w581:dbl, w580:dbl)
          }
          frame 12 {
            n199 = local read "mote12"() -> (w587:cluster{dbl, dbl})
            n200 = Unbundle(w587) -> (w586:dbl, w585:dbl)
          }
          frame 109 {
            n201 = local read "mote109"() -> (w592:cluster{dbl, dbl})
            n202 = Unbundle(w592) -> (w591:dbl, w590:dbl)
          }
          frame 110 {
            n203 = local read "mote110"() -> (w597:cluster{dbl, dbl})
            n204 = Unbundle(w597) -> (w596:dbl, w595:dbl)
          }
          frame 111 {
            n205 = local read "mote111"() -> (w602:cluster{dbl, dbl})
            n206 = Unbundle(w602) -> (w601:dbl, w600:dbl)
          }
        }
        "Temperature" <- w532
        "Humidity" <- w531
        "CO2 Meter" <- w528
        "Light" <- w527
      }
    }
  }
